vi "ReplaceObj.vi"(8 "error in (no error)":errorcluster, 11 "Channel in":refnum<class "Channel.lvclass">) -> (0 "error out":errorcluster, 3 "Channel out":refnum<class "Channel.lvclass">)   [LabVIEW 2018, in "Channel.lvclass"]
uses:
  Channel.lvclass
  Channel.lvclass/Channel.ctl
  Interface/Interface.lvclass
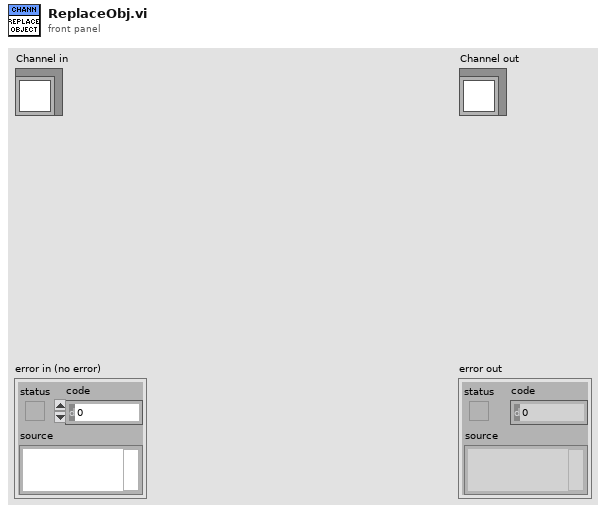
[diagram p1: front panel]
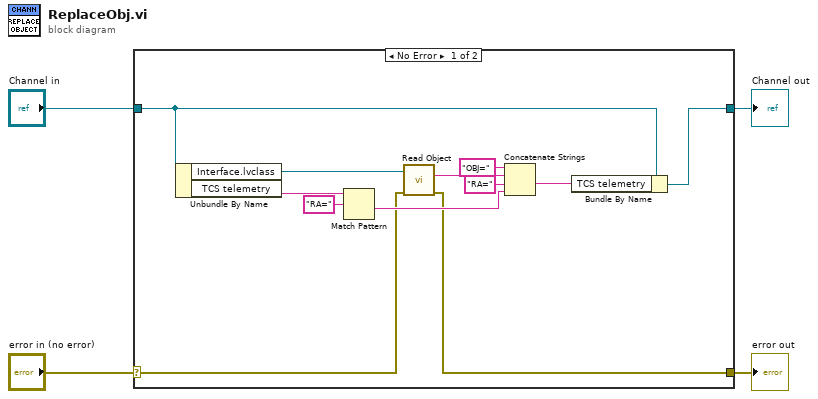
[diagram p0: block diagram]
diagram:
  n1 = case shown="No Error" "error in (no error)" {
    selector: "error in (no error)" -> [w6 w18]
    tunnel: [w5 w18] -> w3
    tunnel: [w7 w17] -> w1
    tunnel: "Channel in" -> [w9 w17]
    frame No Error {
      n2 = Unbundle By Name(w9) -> ("Interface.lvclass"=w14:refnum<class "Interface.lvclass">, "TCS telemetry"=w16:string)
      n3 = Match Pattern(string=w16, regular expression="RA=") -> (after substring=w10:string)  [unwired: 1 in, 3 out]
      n4 = call-dynamic "Read Object.vi"("error in (no error)"=w6, "Interface in"=w14) -> ("error out"=w5:errorcluster, "Object"=w12:string)  [unwired: 7 in, 1 out]
      n5 = Concatenate Strings("OBJ=" ("string"), w12, "RA=" ("string"), w10) -> (w8:string)
      n6 = Bundle By Name(cluster=w9, "TCS telemetry"=w8) -> (w7:refnum<class "Channel.lvclass">)
    }
    frame Error {
    }
  }
  "error out" <- w3
  "Channel out" <- w1
